vi "ziIDToServer.vi"(0 "ziHandle In":T1 {"Handle" format="0x%08x"; "Conn" format="0x%08x"}, 5 "Device ID":string="DEV209", 11 "Error In":errorcluster) -> (4 "ziHandle Out":T1 {"Handle" format="0x%08x"; "Conn" format="0x%08x"}, 6 "ziDiscovery":T2={"timestamp"=0, "deviceid"="", "devicetype"="", "serveraddress"="", "serverport"=0, "apilevel"=0, "discoverable"=TRUE, "interface"="", "connected"="", "available"=TRUE, "owner"="", "status"="", "options "="", "serverversion"=""}, 15 "Error Out":errorcluster)   [LabVIEW 2018, in "Zurich Instruments LabOne.lvlib"]
doc: "Enter the Device ID, e.g., \"DEV2003\", to receive the standard input for ziOpen.vi."
uses:
  Zurich Instruments LabOne.lvlib
  ziTypeDisovery.ctl
  <instrlib>/Zurich Instruments LabOne/Private/ziLV64.framework
  ziTypeHandle.ctl
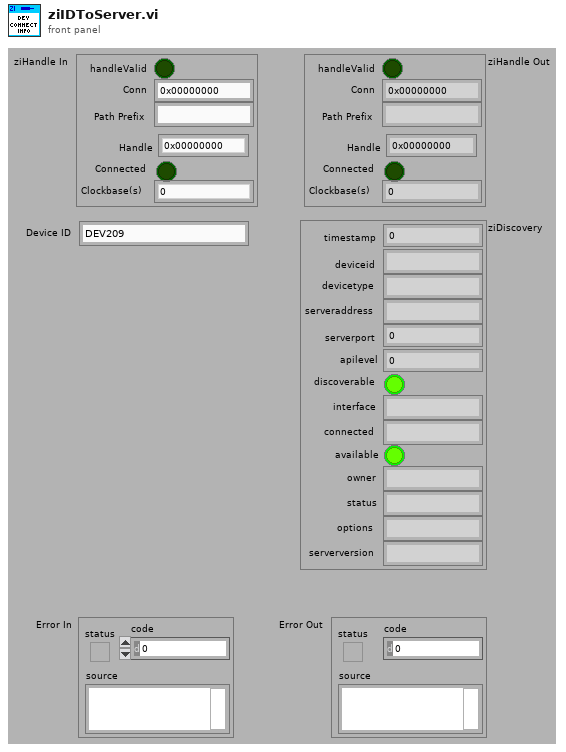
[diagram p1: front panel]
types:
  T1 = typedef "Zurich Instruments LabOne.lvlib/ziTypeHandle.ctl" = cluster{"handleValid":bool, "Conn":u64, "Path Prefix":string, "Handle":u64, "Connected":bool, "Clockbase(s)":dbl}
  T2 = typedef "Zurich Instruments LabOne.lvlib/ziTypeDisovery.ctl" = cluster{"timestamp":u64, "deviceid":string, "devicetype":string, "serveraddress":string, "serverport":u32, "apilevel":u32, "discoverable":bool, "interface":string, "connected":string, "available":bool, "owner":string, "status":string, "options ":string, "serverversion":string}
  T3 = cluster{u64, u8[], u8[], u8[], u32, u32, bool, u8[], u8[], bool, u8[], u8[], u8[], u8[]}
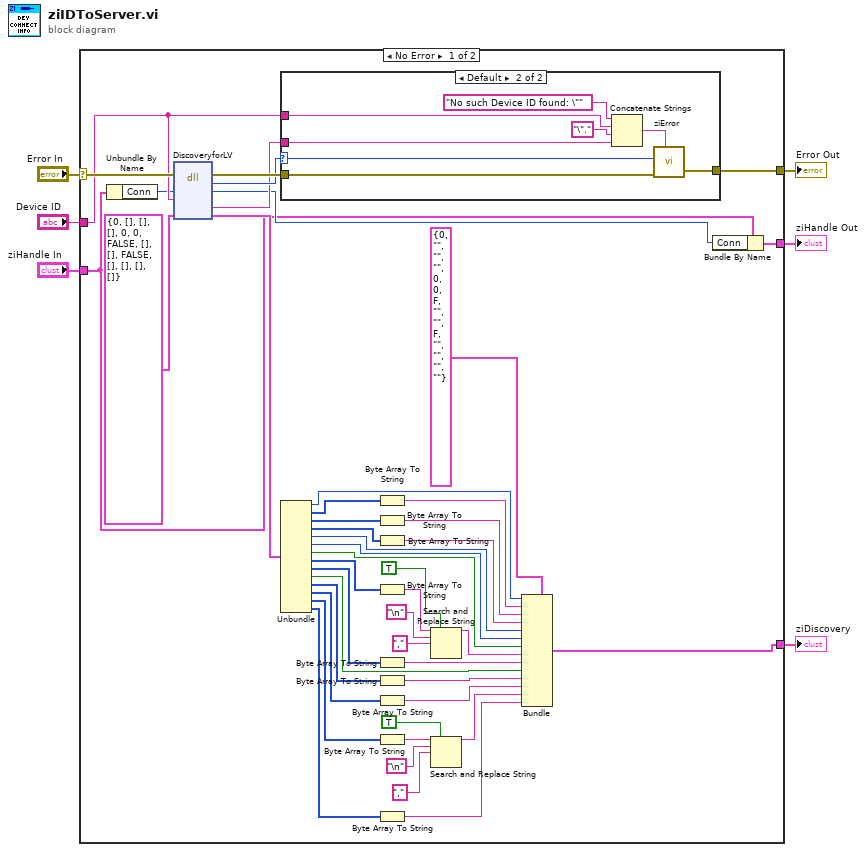
[diagram p0: block diagram]
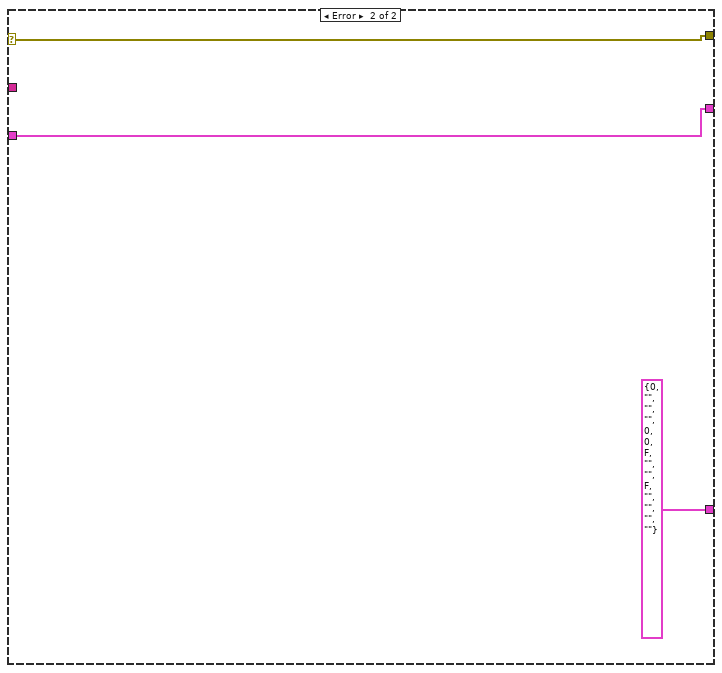
[diagram p3: hidden frame]
diagram:
  n1 = case shown="No Error" "Error In" {
    selector: "Error In" -> [w51 w63]
    tunnel: [w35 w63] -> w4
    tunnel: "Device ID" -> [w49 _]
    tunnel: [w43 T2 {"timestamp"=0, "deviceid"="", "devicetype"="", "serveraddress"="", "serverport"=0, "apilevel"=0, "discoverable"=FALSE, "interface"="", "connected"="", "available"=FALSE, "owner"="", "status"="", "options "="", "serverversion"=""} ("ziDiscoverHandle 2")] -> w3
    tunnel: "ziHandle In" -> [w13 w61]
    tunnel: [w14 w61] -> w1
    frame No Error {
      n2 = Unbundle By Name(w13) -> ("Conn"=w16:u64)
      n3 = dll-call lib="Applications/National Instruments/LabVIEW 2019 64-bit/instr.lib/Zurich Instruments LabOne/Private/ziLV*.*" fn="DiscoveryforLV"(error in=w51, "conn"=w16, "deviceSerial"=w49, "DiscoveryObj"=T3 {0, [], [], [], 0, 0, FALSE, [], [], FALSE, [], [], [], []}) -> (error out=w50:errorcluster, "return type"=w48:u32, "conn"=w15:u64, "ErrorMsg"=w47:string, "DiscoveryObj"=w25:T3)  [unwired: 4 in, 1 out]
      n4 = case shown="Default" w48 {
        selector: w48 -> [_ w54]
        tunnel: w50 -> [w52 w60]
        tunnel: [w52 w59] -> w35
        tunnel: w49 -> [_ w55]
        tunnel: w47 -> [_ w53]
        frame 0 {
        }
        frame Default {
          n5 = Concatenate Strings("No such Device ID found: \"" ("source"), w55, "\"." ("source"), w53) -> (w56:string)
          n6 = call "ziError.vi"("ziErrorCode"=w54, "Error In"=w60, "Annotation"=w56) -> ("Error Out"=w59:errorcluster)  [unwired: 2 in, 1 out]
        }
      }
      n7 = Unbundle(w25) -> (w41:u64, w45:u8[], w44:u8[], w28:u8[], w29:u32, w30:u32, w31:bool, w8:u8[], w33:u8[], w32:bool, w38:u8[], w37:u8[], w26:u8[], w19:u8[])
      n8 = Byte Array To String(unsigned byte array=w45) -> (string=w39:string)
      n9 = Byte Array To String(unsigned byte array=w44) -> (string=w40:string)
      n10 = Byte Array To String(unsigned byte array=w28) -> (string=w27:string)
      n11 = Byte Array To String(unsigned byte array=w8) -> (string=w10:string)
      n12 = Byte Array To String(unsigned byte array=w33) -> (string=w34:string)
      n13 = Byte Array To String(unsigned byte array=w38) -> (string=w36:string)
      n14 = Byte Array To String(unsigned byte array=w37) -> (string=w21:string)
      n15 = Byte Array To String(unsigned byte array=w26) -> (string=w22:string)
      n16 = Byte Array To String(unsigned byte array=w19) -> (string=w18:string)
      n17 = Search and Replace String(replace all?=TRUE ("replace all? (F)"), input string=w10, search string="\n", replace string="," ("replace string (\"\")")) -> (result string=w7:string)  [unwired: 4 in, 3 out]
      n18 = Search and Replace String(replace all?=TRUE ("replace all? (F)"), input string=w22, search string="\n", replace string="," ("replace string (\"\")")) -> (result string=w20:string)  [unwired: 4 in, 3 out]
      n19 = Bundle(cluster=T2 {"timestamp"=0, "deviceid"="", "devicetype"="", "serveraddress"="", "serverport"=0, "apilevel"=0, "discoverable"=FALSE, "interface"="", "connected"="", "available"=FALSE, "owner"="", "status"="", "options "="", "serverversion"=""} ("ziDiscoverHandle 2"), "timestamp"=w41, "deviceid"=w39, "devicetype"=w40, "serveraddress"=w27, "serverport"=w29, "apilevel"=w30, "discoverable"=w31, "interface"=w7, "connected"=w34, "available"=w32, "owner"=w36, "status"=w21, "options"=w20, "serverversion"=w18) -> (w43:T2)
      n20 = Bundle By Name(cluster=w13, "Conn"=w15) -> (w14:T1)
    }
    frame Error {
    }
  }
  "Error Out" <- w4
  "ziDiscovery" <- w3
  "ziHandle Out" <- w1
